vi "New UTF-8 Path.vi"(6 "error in":errorcluster, 9 "LabVIEW Path":T1) -> (1 "UTF-8 Path":refnum<class "UTF-8 Path.lvclass">, 4 "error out":errorcluster)   [LabVIEW 2020, in "G-Unicode.lvlib" / "UTF-8 Path.lvclass"]
doc: "Initializes a new UTF-8 path. <b>LabVIEW Path</b> will be encoded as UTF-8 using the local codepage.\n\nIf you have a LabVIEW path which is already UTF-8 encoded, use <b>Write Raw UTF-8 Path.vi</b> instead."
uses:
  UTF-8 Path.lvclass
  Raw UTF-8 Path.ctl
  UTF-8 Path.lvclass/UTF-8 Path.ctl
  G-Unicode.lvlib
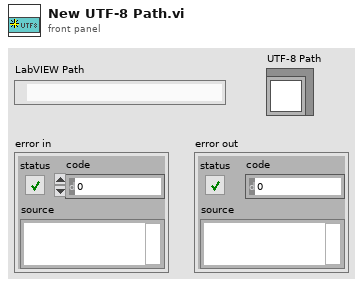
[diagram p1: front panel]
types:
  T1 = typedef "G-Unicode.lvlib/Raw UTF-8 Path.ctl" = path
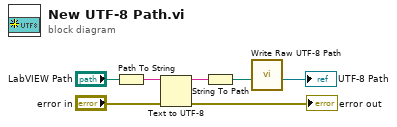
[diagram p0: block diagram]
diagram:
  n1 = Path To String(path="LabVIEW Path") -> (string=w4:string)
  n2 = Text to UTF-8(8:"error in", 11:w4) -> (0:→"error out":errorcluster, 3:w3:string)  [unwired: 1 in]
  n3 = String To Path(string=w3) -> (path=w2:path)
  n4 = call "Write Raw UTF-8 Path.vi"("Raw UTF-8 Path"=w2) -> ("UTF-8 Path"=→"UTF-8 Path":refnum<class "UTF-8 Path.lvclass">)  [unwired: 10 in]
